vi "Set Module Config.vi"(8 "error in (no error)":errorcluster, 10 "Config Channels":dbl[](array[numeric]), 11 "9235 in":refnum<class "9235.lvclass">) -> (0 "error out":errorcluster, 3 "9235 out":refnum<class "9235.lvclass">)   [LabVIEW 2020, in "Modules.lvlib" / "9235.lvclass"]
uses:
  9235.lvclass
  9235.lvclass/9235.ctl
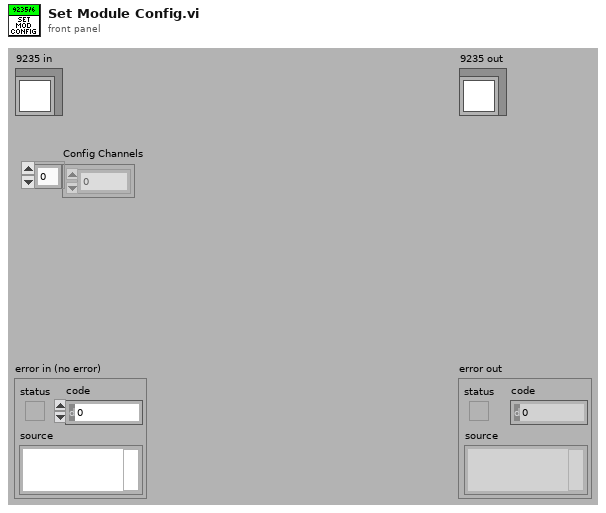
[diagram p1: front panel]
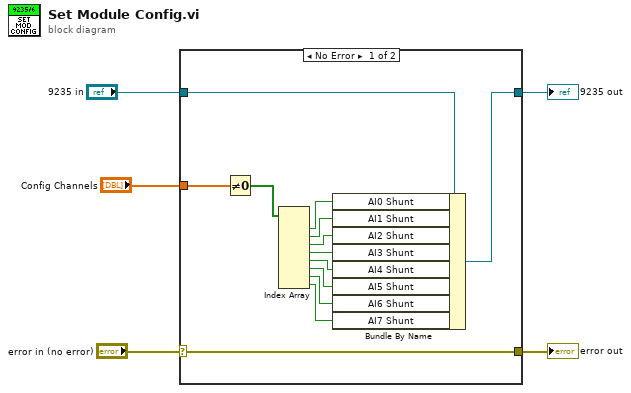
[diagram p0: block diagram]
diagram:
  n1 = case shown="No Error" "error in (no error)" {
    selector: "error in (no error)" -> [w10 w20]
    tunnel: "9235 in" -> [w18 w19]
    tunnel: "Config Channels" -> [w17 _]
    tunnel: [w10 w20] -> w2
    tunnel: [w11 w19] -> w1
    frame No Error {
      n2 = Not Equal To 0?(x=w17) -> (x != 0?=w16:bool[])
      n3 = Index Array(array=w16) -> (element #1=w15:bool, element #2=w14:bool, element #3=w13:bool, element #4=w12:bool, element #5=w9:bool, element #6=w8:bool, element #7=w7:bool, element #8=w6:bool)  [unwired: 8 in]
      n4 = Bundle By Name(cluster=w18, "AI0 Shunt"=w15, "AI1 Shunt"=w14, "AI2 Shunt"=w13, "AI3 Shunt"=w12, "AI4 Shunt"=w9, "AI5 Shunt"=w8, "AI6 Shunt"=w7, "AI7 Shunt"=w6) -> (w11:refnum<class "9235.lvclass">)
    }
    frame Error {
    }
  }
  "error out" <- w2
  "9235 out" <- w1
